vi "Add.vi"(8 "error in (no error)":errorcluster, 9 "Name":string, 10 "LabVIEW Object":refnum<class>, 11 "Collection in":refnum<class "CollectionByValue.lvclass">) -> (0 "error out":errorcluster, 3 "Collection out":refnum<class "CollectionByValue.lvclass">)   [LabVIEW 2021, in "Collection.lvlib" / "CollectionByValue.lvclass"]
uses:
  CollectionByValue.lvclass
  CollectionByValue.lvclass/CollectionByValue.ctl
panel:
  # "PRivate"
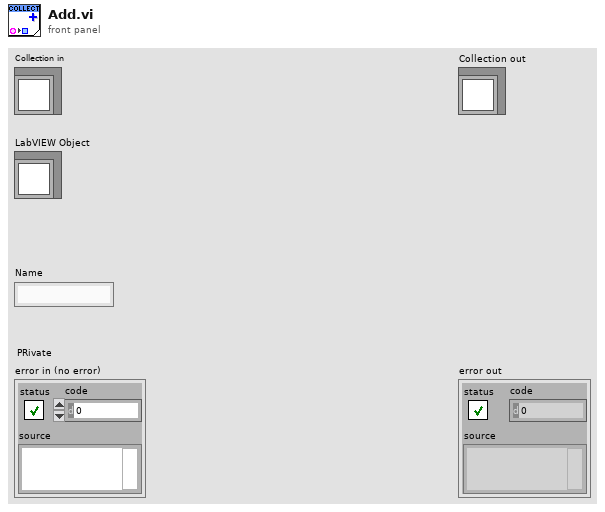
[diagram p1: front panel]
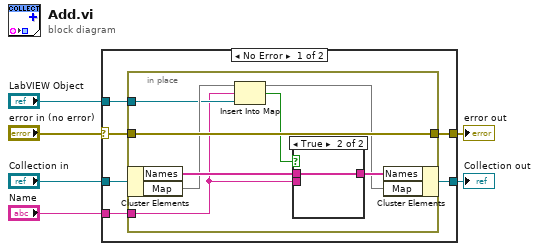
[diagram p0: block diagram]
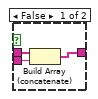
[diagram p2: hidden frame]
diagram:
  n1 = case shown="No Error" "error in (no error)" {
    selector: "error in (no error)" -> [w11 w26]
    tunnel: [w10 w26] -> w5
    tunnel: [w7 w25] -> w3
    tunnel: "Collection in" -> [w8 w25]
    tunnel: "LabVIEW Object" -> [w12 _]
    tunnel: "Name" -> [w9 _]
    frame No Error {
      n2 = in-place {
        in-place-border: w12 -> [w15]
        in-place-border: w11 -> [w18]
        in-place-border: [w18] -> w10
        in-place-border: w9 -> [w14]
        n3 = in-place-cluster #1(w8) -> ("Names"=w20:string[], "Map"=w17:map{string, refnum<class>})
        n4 = Insert Into Map(map in=w17, key=w14, value=w15) -> (map out=w16:map{string, refnum<class>}, key already included?=w13:bool)  [unwired: 1 out]
        n5 = case shown="True" w13 {
          tunnel: w20 -> [w23 w24]
          tunnel: [w22 w24] -> w19
          tunnel: w14 -> [w21 _]
          frame False {
            n6 = Build Array (concatenate)(w23, w21) -> (w22:string[])
          }
          frame True {
          }
        }
        n7 = in-place-cluster #1("Names"=w19, "Map"=w16) -> (w7:refnum<class "CollectionByValue.lvclass">)
      }
    }
    frame Error {
    }
  }
  "error out" <- w5
  "Collection out" <- w3
